vi "SUB_Telnet_READ_FindString.vi"(9 "Find this String":string, 10 "timeout ms":i32=25000, 11 "telnet connection":T1) -> (1 "MSG OUT":string, 2 "Found":bool, 3 "telnet connection out":T1)   [LabVIEW 2011]
uses:
  <vilib>/addons/internet/telnet/telnet.llb/Telnet Session.ctl
  <vilib>/addons/internet/NI_InternetTK_Core_VIs.lvlib
panel:
  out "error out":errorcluster
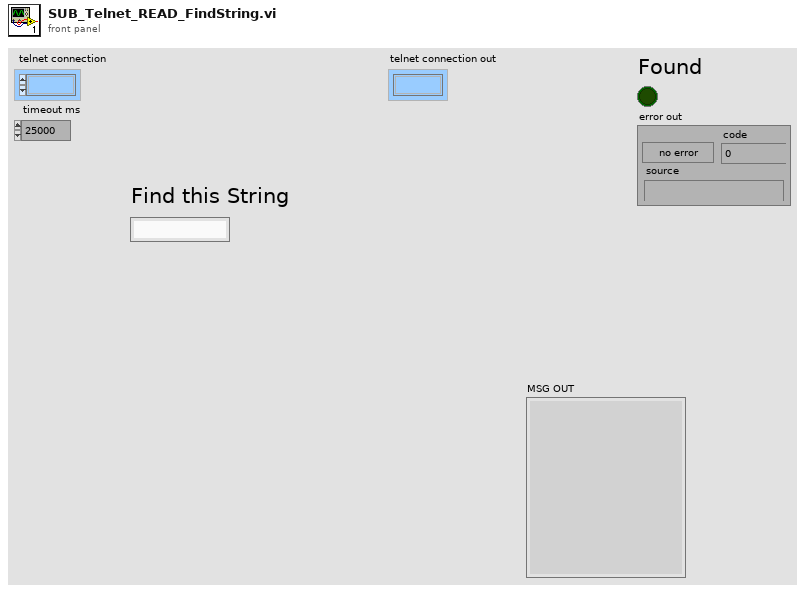
[diagram p1: front panel]
types:
  T1 = typedef "Telnet Session.ctl" = refnum<k1>
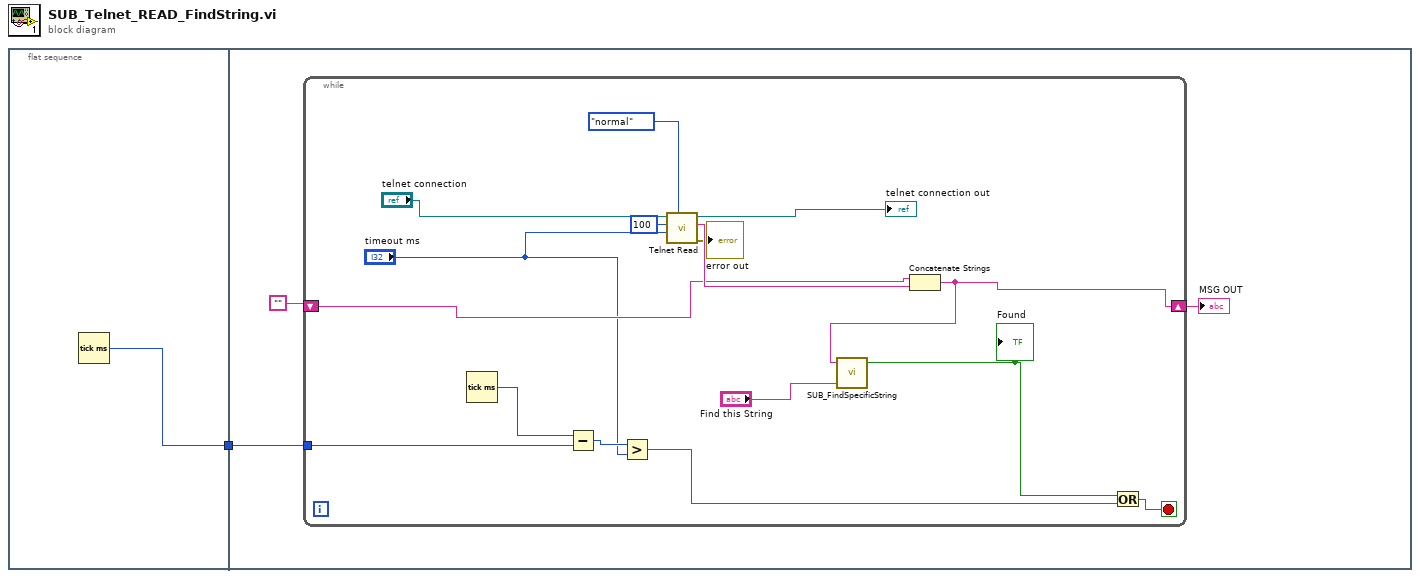
[diagram p0: block diagram]
diagram:
  n1 = flat-sequence {
    tunnel: [w2] -> w1
    tunnel: w1 -> [w4]
    frame #0 {
      n2 = Tick Count (ms)() -> (millisecond timer value=w2:u32)
    }
    frame #1 {
      n3 = while {
        shift-right: [w6] -> w3
        shift-left: "" -> [w17]
        tunnel: w4 -> [w15]
        stop <- w12 stop-if-true
        n4 = Tick Count (ms)() -> (millisecond timer value=w16:u32)
        n5 = Subtract(x=w16, y=w15) -> (x-y=w14:u32)
        n6 = Greater?(x=w14, y="timeout ms") -> (0:w10:bool)
        n7 = call <vilib>:"Telnet Read.vi"("read mode (normal)"=enum16{"normal", "line", "buffered"}."normal", "timeout ms (25000)"="timeout ms", "bytes to read"=100, "telnet connection"="telnet connection") -> ("error out"=→"error out":errorcluster, "data out"=w18:string, "telnet connection out"=→"telnet connection out":T1)  [unwired: 3 in]
        n8 = Concatenate Strings(w17, w18) -> (w6:string)
        n9 = call "SUB_FindSpecificString.vi"("Find this String"="Find this String", "String data"=w6) -> ("Found"=w11:bool)  [unwired: 2 in, 1 out]
        "Found" <- w11
        n10 = Or(x=w11, y=w10) -> (x .or. y?=w12:bool)
      }
      "MSG OUT" <- w3
    }
  }
